vi "create test taglist.vi"(11 "count":i32=5000) -> (0 "indices":i32[](array[numeric]), 1 "types":T1[](array[typedef]), 2 "names/metadata":string[](array[string]), 3 "tags":refnum<class "data bus tag description.lvclass">[](array[class]))   [LabVIEW 2013, in "tag bus tests.lvlib"]
uses:
  tag bus tests.lvlib
  tag/data bus tag description.lvclass
  tag/Data Type.ctl
  tag/data bus tag description.lvclass/data bus tag description.ctl
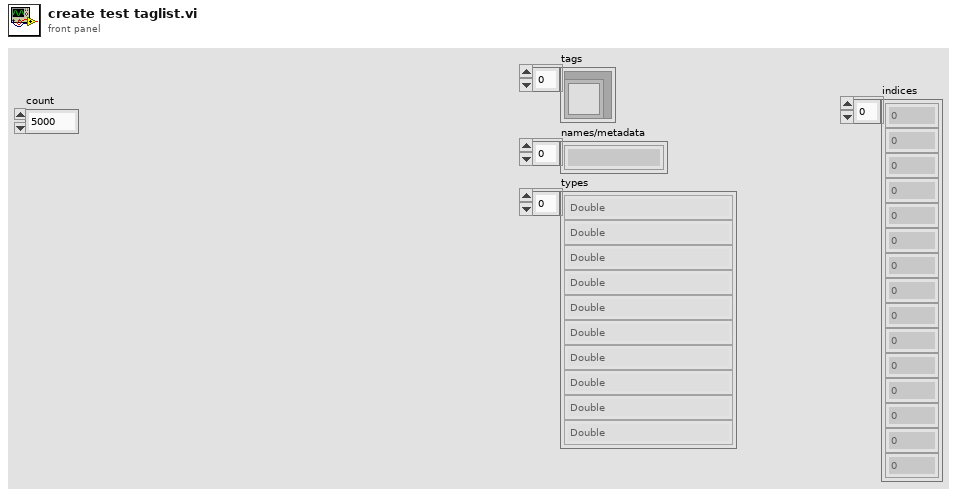
[diagram p1: front panel]
types:
  T1 = typedef "data bus tag description.lvclass/Data Type.ctl" = enum16{"Double", "I64", "Boolean", "Array of Double", "Array of I64", "Variant"}
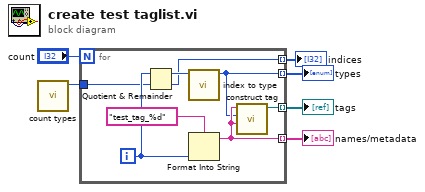
[diagram p0: block diagram]
diagram:
  n1 = call "count types.vi"() -> ("type count"=w5:i32)  [unwired: 11 in]
  n2 = for {
    N: "count" -> [_]
    tunnel: [w14] -> w6 mode=indexing
    tunnel: w5 -> [w11]
    tunnel: [w9] -> w4 mode=indexing
    tunnel: [w8] -> w3 mode=indexing
    tunnel: [w7] -> w1 mode=indexing
    i -> [w12]
    n3 = Quotient & Remainder(x=w12, y=w11) -> (x-y*floor(x/y)=w10:i32, floor(x/y)=w7:i32)
    n4 = call "index to type.vi"("I32"=w10) -> ("type"=w8:T1)  [unwired: 10 in]
    n5 = Format Into String(format string="test_tag_%d", w12) -> (resulting string=w9:string)  [unwired: 2 in, 1 out]
    n6 = call "construct tag.vi"("metadata"=w9, "data type"=w8, "name"=w9) -> ("system tag out"=w14:refnum<class "data bus tag description.lvclass">)  [unwired: 8 in]
  }
  "tags" <- w6
  "names/metadata" <- w4
  "types" <- w3
  "indices" <- w1
